vi "Display Timeout Two Button Popup (SVG).vi"(4 "Message Size":T1={"Message Height"=-1, "Message Width"=-1, "Message Location"=enum."Bottom"} {"Message Width" min=-1 step=1; "Message Height" min=-1 step=1}, 5 "N-Text":string="No", 6 "Theme":refnum<class "Theme.lvclass">, 7 "Y-Text":string="Yes", 8 "Error In":errorcluster, 9 "Timeout (s)":dbl=1.0, 10 "Message":string, 11 "Graphic":path) -> (0 "Error Out":errorcluster, 1 "Choice?":bool, 2 "Timeout":bool)   [LabVIEW 2021, in "SVG - Timeout Two Button.lvclass"]
doc: "The custom two button popup will display information to the user and wait for the operator to click a button or until time expires.\n\n<b>Note:</b> This popup type allows the user to define a custom image for the display. The developer should test all settings prior to deployment to make sure that all images and text fit on the screen correctly.\n\n<b>Note:</b> The function <b>Close Pop-Up (Two Button Choice).vi</b> can be used to send a value when closing this dialog. Otherwise, use Close Pop-Up.vi to close early.\n\nInputs:\n-Graphic [path] - path to the image file to display\n-Message [String] - String Variable to populate Display with\n-Theme [lvclass] - the theme for the style of the popup\n-Message Info [typedef enum]\n -Message Height [I32] - the height for the message text box (-1 = match height of image)\n -Message Width [I32] - the width for the message text box (-1 = match height of image)\n -Message Location [Ring] - the location of the image relative to the message text box (left,\n right,bottom, top)\n-YText [string] - the string for the YES button\n-NText [string] - the string for the NO button\n-Timeout (s) [DBL] - the timeout duration\n\nOutputs\n-Choice? [Boolean] - the user select (YText = True, NText = False)\n\n<b>Code Developed By:</b>\nDaniel Coons\nTechnology Service Corporation\n1983 S Liberty Drive\nBloomington, IN 47403\nPhone: 812 558-7100\ndaniel.coons@tsc.com\nwww.tsc.com/atcs"
uses:
  SVG - Timeout Two Button.lvclass
  SVG - Timeout Two Button.lvclass/SVG - Timeout Two Button.ctl
  <vilib>/addons/_TSC/TSC Pop-Up/Popup/Popup.lvclass
  C:/Development/tsc-pop-up-svg/SVG Parent.lvclass
  C:/Program Files (x86)/National Instruments/LabVIEW 2021/vi.lib/addons/_TSC/TSC Pop-Up/Popup/Popup.lvclass
  C:/Development/tsc-pop-up-svg/Custom/SVG - Timeout Two Button/SVG - Timeout Two Button.lvclass
  <vilib>/addons/_TSC/TSC Pop-Up/Popup/message info--typedef.ctl
  <vilib>/addons/_TSC/TSC Pop-Up/Theme/Theme.lvclass
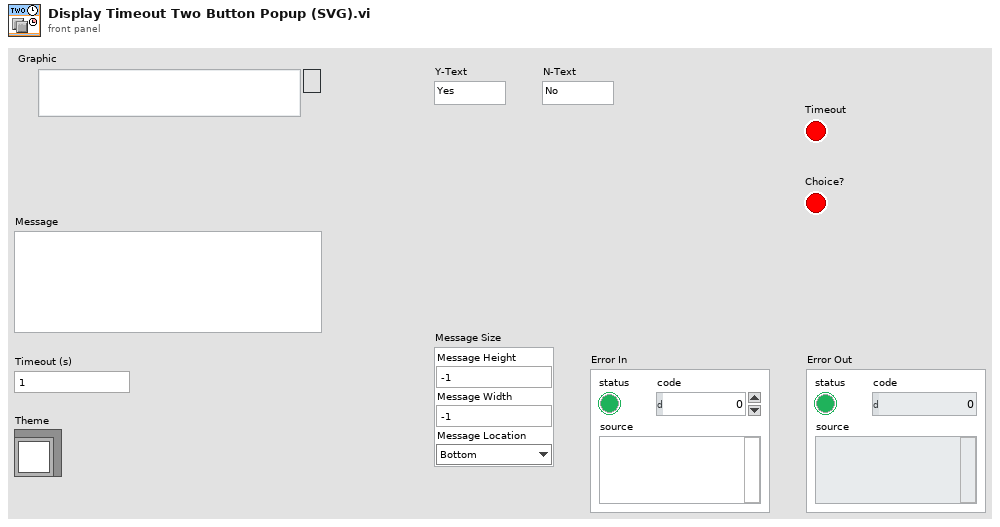
[diagram p1: front panel]
types:
  T1 = typedef "Pop-Up.lvlib/Popup.lvclass/message info--typedef.ctl" = cluster{"Message Height":i32, "Message Width":i32, "Message Location":enum16{"Top", "Bottom", "Right", "Left"}}
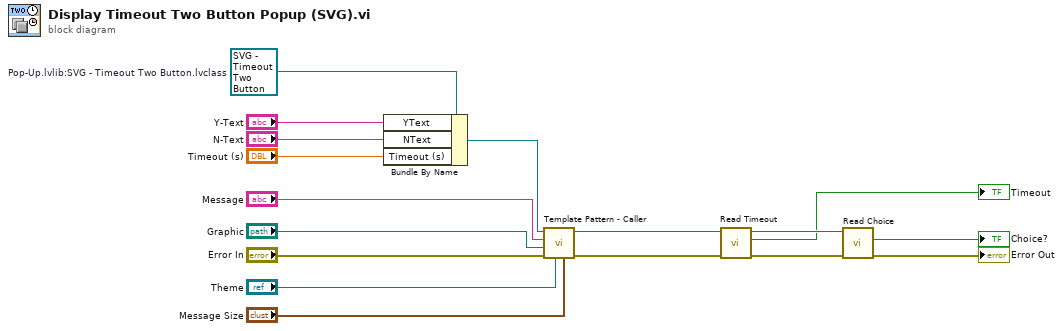
[diagram p0: block diagram]
diagram:
  w8 = refnum<class "SVG - Timeout Two Button.lvclass"> refnum  # Pop-Up.lvlib:SVG - Timeout Two Button.lvclass
  n1 = Bundle By Name(cluster=w8, "YText"="Y-Text", "NText"="N-Text", "Timeout (s)"="Timeout (s)") -> (w9:refnum<class "SVG - Timeout Two Button.lvclass">)
  n2 = call-dynamic "Template Pattern - Caller.vi"("Message Size"="Message Size", "Theme"="Theme", "error in (no error)"="Error In", "Graphic"="Graphic", "Message"="Message", "Pop-Up in"=w9) -> ("error out"=w10:errorcluster, "Pop-Up out"=w3:refnum<class "SVG - Timeout Two Button.lvclass">)  [unwired: 4 in]
  n3 = call <vilib>:"Read Timeout.vi"("error in (no error)"=w10, "Popup in"=w3) -> ("error out"=w4:errorcluster, "Timeout?"=→"Timeout":bool, "Popup in"=w2:refnum<class "SVG - Timeout Two Button.lvclass">)  [unwired: 7 in]
  n4 = call-dynamic "Read Choice.vi"("error in (no error)"=w4, "_Popup in"=w2) -> ("error out"=→"Error Out":errorcluster, "Choice"=→"Choice?":bool)  [unwired: 7 in, 1 out]
